vi "bcd_counter.vi"(0 "bcd":u8[](array[numeric])) -> (4 "decimal":i32)   [LabVIEW 2019]
doc: "Convert a bcd encoded array to its decimal representation"
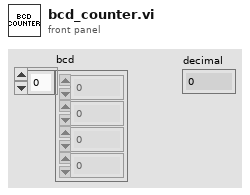
[diagram p1: front panel]
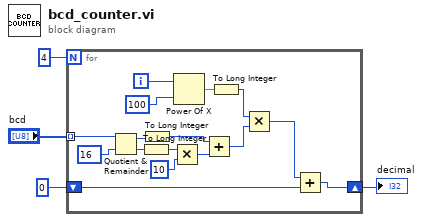
[diagram p0: block diagram]
diagram:
  n1 = for {
    N: 4 -> [_]
    tunnel: "bcd" -> [w20] mode=indexing
    shift-right: [w5] -> w1
    shift-left: 0 ("decimal") -> [w7]
    i -> [w12]
    n2 = Quotient & Remainder(x=w20, y=u8 16) -> (x-y*floor(x/y)=w14:u8, floor(x/y)=w18:u8)
    n3 = To Long Integer(number=w18) -> (32bit integer=w17:i32)
    n4 = To Long Integer(number=w14) -> (32bit integer=w13:i32)
    n5 = Multiply(x=w17, y=10 ("decimal")) -> (x*y=w15:i32)
    n6 = Power Of X(1:100 ("decimal"), 2:w12) -> (0:w10:dbl)
    n7 = Add(x=w13, y=w15) -> (x+y=w8:i32)
    n8 = To Long Integer(number=w10) -> (32bit integer=w9:i32)
    n9 = Multiply(x=w9, y=w8) -> (x*y=w6:i32)
    n10 = Add(x=w6, y=w7) -> (x+y=w5:i32)
  }
  "decimal" <- w1
